vi "DT3120_SetInputSource.vi"(8 "error in (no error)":errorcluster, 10 "NewSource":u16, 11 "DevId":i32) -> (0 "error out":errorcluster, 2 "Old Source":u16, 3 "DevId (dup)":i32)   [LabVIEW 2009]
uses:
  olfg32.dll
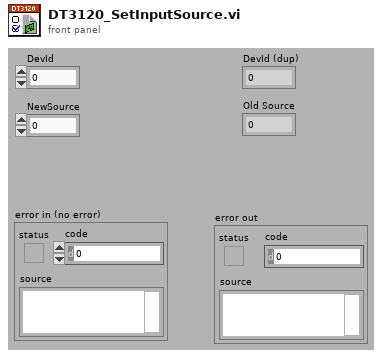
[diagram p1: front panel]
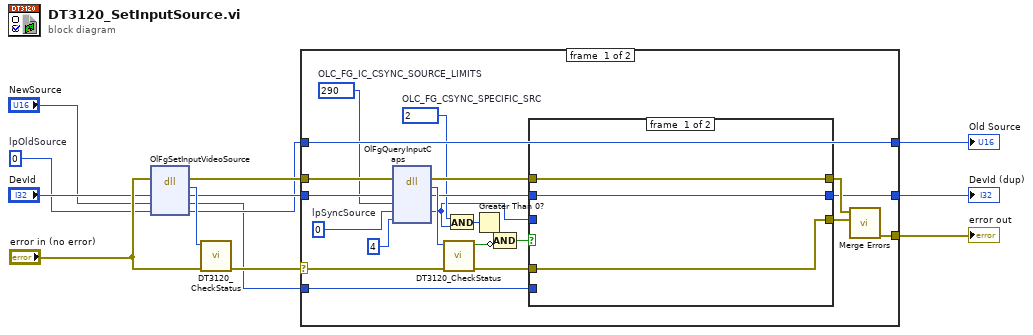
[diagram p0: block diagram]
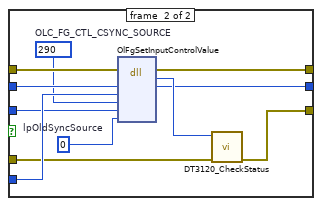
[diagram p2: hidden frame]
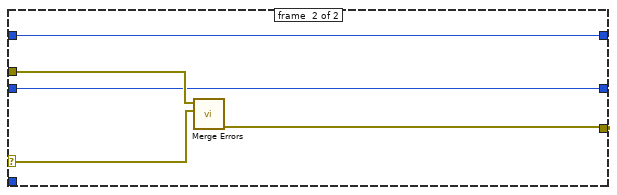
[diagram p3: hidden frame]
diagram:
  w8 = u16 0  # lpOldSource
  n1 = dll-call lib="C:/LabVIEW Programs/MT Scan/SubVIs/olfg32.dll" fn="OlFgSetInputVideoSource"(error in="error in (no error)", "DevId"="DevId", "NewSource"="NewSource", "lpOldSource"=w8) -> (error out=w11:errorcluster, "Status"=w10:u32, "DevId"=w6:i32, "NewSource"=w1:u16, "lpOldSource"=w2:u16)  [unwired: 2 in, 1 out]
  n2 = call "DT3120_CheckStatus.vi"("error in"="error in (no error)", "Status"=w10) -> ("error out"=w7:errorcluster)  [unwired: 9 out]
  n3 = case shown="No Error" w7 {
    selector: w7 -> [w34 w52]
    tunnel: w11 -> [w33 w53]
    tunnel: [w35 w54] -> w13
    tunnel: w6 -> [w31 w51]
    tunnel: [w14 w51] -> w5
    tunnel: [w29 w50] -> w4
    tunnel: w2 -> [w29 w50]
    tunnel: w1 -> [w18 _]
    frame #0 {
      w21 = u32 2  # OLC_FG_CSYNC_SPECIFIC_SRC
      w28 = 290  # OLC_FG_IC_CSYNC_SOURCE_LIMITS
      w30 = u32 0  # lpSyncSource
      n4 = dll-call lib="C:/LabVIEW Programs/MT Scan/SubVIs/olfg32.dll" fn="OlFgQueryInputCaps"(error in=w33, "DevId"=w31, "Key"=w28, "lpData"=w30, "DataSize"=u32 4) -> (error out=w25:errorcluster, "Status"=w32:u32, "DevId"=w24:i32, "lpData"=w17:u32)  [unwired: 4 in, 1 out]
      n5 = call "DT3120_CheckStatus.vi"("error in"=w34, "Status"=w32) -> ("error out"=w26:errorcluster, "New Error?"=w22:bool)  [unwired: 2 in, 6 out]
      n6 = And(x=w21, y=w17) -> (x .and. y?=w20:u32)
      n7 = Greater Than 0?(x=w20) -> (x > 0?=w19:bool)
      n8 = Compound Arithmetic op=AND(w19, invert w22) -> (w23:bool)
      n9 = case shown="True" w23 {
        tunnel: w26 -> [w37 w43]
        tunnel: w25 -> [w38 w49]
        tunnel: w24 -> [w36 w48]
        tunnel: w18 -> [_ w47]
        tunnel: w17 -> [_ w44]
        tunnel: [w37 w42] -> w16
        tunnel: [w38 w40] -> w15
        tunnel: [w36 w39] -> w14
        frame #0 {
        }
        frame #1 {
          w45 = 290  # OLC_FG_CTL_CSYNC_SOURCE
          w46 = u32 0  # lpOldSyncSource
          n10 = dll-call lib="C:/LabVIEW Programs/MT Scan/SubVIs/olfg32.dll" fn="OlFgSetInputControlValue"(error in=w49, "DevId"=w48, "Source"=w47, "Control"=w45, "NewData"=w44, "lpOldData"=w46) -> (error out=w40:errorcluster, "Status"=w41:u32, "DevId"=w39:i32)  [unwired: 5 in, 2 out]
          n11 = call "DT3120_CheckStatus.vi"("error in"=w43, "Status"=w41) -> ("error out"=w42:errorcluster)  [unwired: 2 in, 7 out]
        }
      }
      n12 = call <vilib>:"Merge Errors.vi"("error in 2 (no error)"=w16, "error in 1 (no error)"=w15) -> ("error out"=w35:errorcluster)  [unwired: 2 in, 3 out]
    }
    frame #1 {
      n13 = call <vilib>:"Merge Errors.vi"("error in 2 (no error)"=w52, "error in 1 (no error)"=w53) -> ("error out"=w54:errorcluster)  [unwired: 2 in, 3 out]
    }
  }
  "error out" <- w13
  "DevId (dup)" <- w5
  "Old Source" <- w4
